vi "Cheesy_drive.vi"(5 "Speedturn_Sens_Low max":dbl=0.6, 6 "Quickturn_Sens_Low":dbl=1.0, 7 "Speedturn_Sens_Low":dbl=0.6, 9 "Quick Turn":bool, 10 "Wheel":dbl, 11 "Throttle":dbl) -> (3 "Drive Data":cluster{"Left":dbl, "Right":dbl})   [LabVIEW 2015]
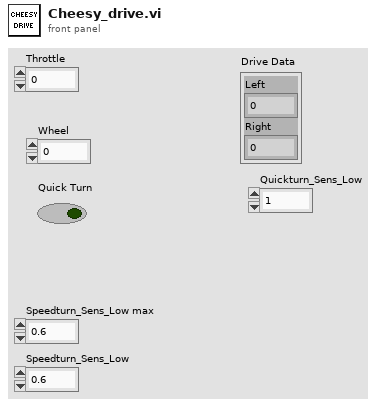
[diagram p1: front panel]
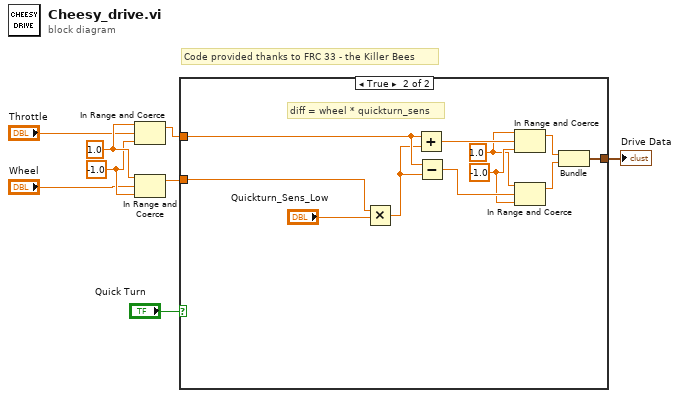
[diagram p0: block diagram]
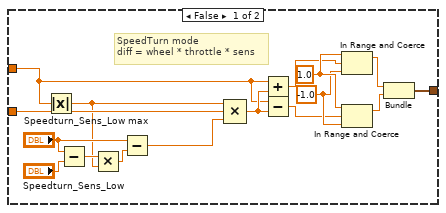
[diagram p2: hidden frame]
diagram:
  w5 = -1.0 ("lower limit")
  w6 = 1.0 ("upper limit")
  # "Code provided thanks to FRC 33 - the Killer Bees"
  n1 = In Range and Coerce(upper limit=w6, x="Throttle", lower limit=w5) -> (coerced(x)=w3:dbl)  [unwired: 1 out]
  n2 = In Range and Coerce(upper limit=w6, x="Wheel", lower limit=w5) -> (coerced(x)=w4:dbl)  [unwired: 1 out]
  n3 = case shown="True" "Quick Turn" {
    tunnel: w4 -> [w24 w35]
    tunnel: w3 -> [w18 w34]
    tunnel: [w10 w32] -> w8
    frame False {
      w15 = -1.0 ("lower limit")
      w16 = 1.0 ("upper limit")
      # "SpeedTurn mode\ndiff = wheel * throttle * sens"
      n4 = Absolute Value(x=w18) -> (abs(x)=w17:dbl)
      n5 = Subtract(x="Speedturn_Sens_Low max", y="Speedturn_Sens_Low") -> (x-y=w21:dbl)
      n6 = Multiply(x=w21, y=w17) -> (x*y=w19:dbl)
      n7 = Subtract(x="Speedturn_Sens_Low max", y=w19) -> (x-y=w9:dbl)
      n8 = Compound Arithmetic op=MULTIPLY(w17, w24, w9) -> (w23:dbl)
      n9 = Add(x=w18, y=w23) -> (x+y=w14:dbl)
      n10 = Subtract(x=w18, y=w23) -> (x-y=w13:dbl)
      n11 = In Range and Coerce(upper limit=w16, x=w14, lower limit=w15) -> (coerced(x)=w11:dbl)  [unwired: 1 out]
      n12 = In Range and Coerce(upper limit=w16, x=w13, lower limit=w15) -> (coerced(x)=w12:dbl)  [unwired: 1 out]
      n13 = Bundle("upper limit"=w11, "upper limit"=w12) -> (w10:cluster{"upper limit":dbl, "upper limit":dbl})  [unwired: 1 in]
    }
    frame True {
      w27 = -1.0 ("lower limit")
      w26 = 1.0 ("upper limit")
      # "diff = wheel * quickturn_sens"
      n14 = Multiply(x=w35, y="Quickturn_Sens_Low") -> (x*y=w33:dbl)
      n15 = Add(x=w34, y=w33) -> (x+y=w31:dbl)
      n16 = Subtract(x=w34, y=w33) -> (x-y=w29:dbl)
      n17 = In Range and Coerce(upper limit=w26, x=w31, lower limit=w27) -> (coerced(x)=w30:dbl)  [unwired: 1 out]
      n18 = In Range and Coerce(upper limit=w26, x=w29, lower limit=w27) -> (coerced(x)=w28:dbl)  [unwired: 1 out]
      n19 = Bundle("upper limit"=w30, "upper limit"=w28) -> (w32:cluster{"upper limit":dbl, "upper limit":dbl})  [unwired: 1 in]
    }
  }
  "Drive Data" <- w8
